vi "Format String To Format Code.vi"(11 "Start String":string) -> (0 "Error":bool, 1 "Format Code":T1, 2 "Delim":string, 3 "Remaining String":string)   [LabVIEW 2018, in "Numeric Data Type.lvclass"]
uses:
  Numeric Data Type.lvclass
  Format Code.ctl
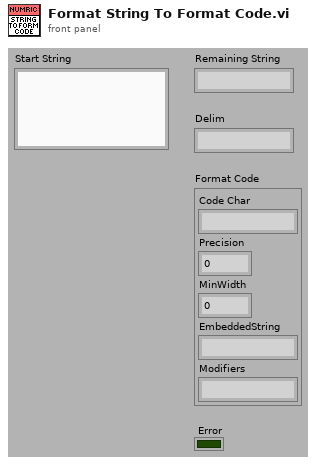
[diagram p1: front panel]
types:
  T1 = typedef "Numeric Data Type.lvclass/Format Code.ctl" = cluster{"Code Char":string, "Precision":i32, "MinWidth":u16, "EmbeddedString":string, "Modifiers":string}
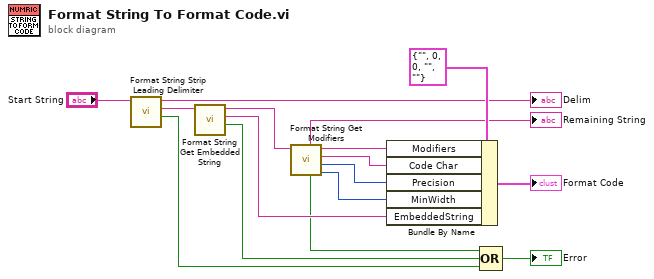
[diagram p0: block diagram]
diagram:
  n1 = call "Format String Strip Leading Delimiter.vi"("Start String"="Start String") -> ("Error"=w12:bool, "Remaining String"=w11:string, "Delim"=→"Delim":string)  [unwired: 8 in]
  n2 = call "Format String Get Embedded String.vi"("Start String"=w11) -> ("Error"=w9:bool, "EmbeddedString"=w10:string, "Remaining String"=w8:string)  [unwired: 8 in]
  n3 = call "Format String Get Modifiers.vi"("Start String"=w8) -> ("Min Width"=w3:u16, "Precision"=w4:i32, "Code Character"=w5:string, "Modifiers"=w6:string, "Error"=w2:bool, "Remaining String"=→"Remaining String":string)  [unwired: 5 in]
  n4 = Bundle By Name(cluster=T1 {"Code Char"="", "Precision"=0, "MinWidth"=0, "EmbeddedString"="", "Modifiers"=""} ("FormatCode"), "Modifiers"=w6, "Code Char"=w5, "Precision"=w4, "MinWidth"=w3, "EmbeddedString"=w10) -> (→"Format Code":T1)
  n5 = Compound Arithmetic op=OR(w2, w9, w12) -> (→"Error":bool)
